vi "AssertsVIExecStateNotBadorRun.vi"(0 "VI Reference In":refnum<vi>, 1 "Label (VI Title)":string="Default", 11 "error in":errorcluster) -> (4 "VI Reference Out":refnum<vi>, 15 "error out":errorcluster)   [LabVIEW 2016, in "DronaTest.lvlib"]
uses:
  DronaTest.lvlib
  APIs/Assert/AssertVI/AssertVIExecRunning.vi
  <vilib>/addons/_JKI Toolkits/Caraya/classes/Assert/Assert Not Error.vi
  APIs/Assert/AssertVI/AssertVIExecNotBad.vi
  APIs/Assert/AssertVI/AssertVIExecBad.vi
  <vilib>/addons/_JKI Toolkits/Caraya/classes/Assert/Assert Error.vi
  <vilib>/addons/_JKI Toolkits/Caraya/classes/Test/Test.lvclass
  Drona.lvlib
  <vilib>/addons/_JKI Toolkits/Caraya/classes/Assert/Assert.lvclass
  APIs/Assert/AssertVI/AssertVI.lvlib
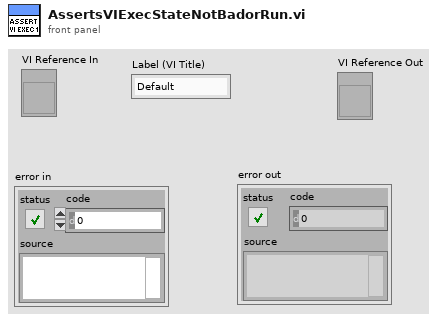
[diagram p1: front panel]
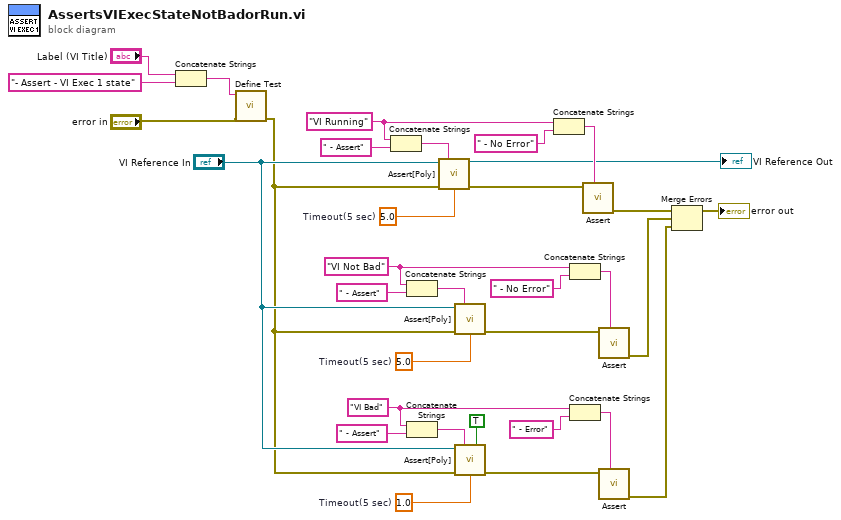
[diagram p0: block diagram]
diagram:
  w9 = "VI Bad" ("Label")
  w6 = 1.0  # Timeout(5 sec)
  w17 = "VI Not Bad" ("Label")
  w20 = 5.0  # Timeout(5 sec)
  w27 = "VI Running" ("Label")
  w24 = 5.0  # Timeout(5 sec)
  n1 = Concatenate Strings("Label (VI Title)", "- Assert - VI Exec 1 state" ("string")) -> (w31:string)
  n2 = call <vilib>:"Define Test.vi"("error in (no error)"="error in", "Label (VI Title)"=w31) -> ("error out"=w3:errorcluster)  [unwired: 9 in]
  n3 = Concatenate Strings(w27, " - Assert" ("string")) -> (w25:string)
  n4 = Concatenate Strings(w17, " - Assert" ("string")) -> (w19:string)
  n5 = Concatenate Strings(w9, " - Assert" ("string")) -> (w7:string)
  n6 = call-poly "Assert[Poly].vi"("VI Reference In"="VI Reference In", "Test Label"=w25, "Error In"=w3, "Timeout(5 sec)"=w24) -> ("VI Reference Out"=→"VI Reference Out":refnum<vi>, "Error Out"=w22:errorcluster)  [unwired: 10 in]
  n7 = call-poly "Assert[Poly].vi"("VI Reference In"="VI Reference In", "Test Label"=w19, "Error In"=w3, "Timeout(5 sec)"=w20) -> ("Error Out"=w21:errorcluster)  [unwired: 10 in, 1 out]
  n8 = call-poly "Assert[Poly].vi"("VI Reference In"="VI Reference In", "Label"=w7, "Assert Only? (F)"=TRUE, "Error In"=w3, "Timeout(5 sec)"=w6) -> ("Error Out"=w5:errorcluster)  [unwired: 9 in, 1 out]
  n9 = Concatenate Strings(w27, " - No Error" ("string")) -> (w33:string)
  n10 = Concatenate Strings(w17, " - No Error" ("string")) -> (w15:string)
  n11 = Concatenate Strings(w9, " - Error" ("string")) -> (w11:string)
  n12 = call-poly <vilib>:"Assert.vi"("Label"=w33, "Not Error?"=w22) -> ("error out"=w13:errorcluster)  [unwired: 9 in]
  n13 = call-poly <vilib>:"Assert.vi"("Label"=w15, "Not Error?"=w21) -> ("error out"=w14:errorcluster)  [unwired: 9 in]
  n14 = call-poly <vilib>:"Assert.vi"("Label"=w11, "Error?"=w5) -> ("error out"=w1:errorcluster)  [unwired: 9 in]
  n15 = Merge Errors(w13, w14, w1) -> (→"error out":errorcluster)
